vi "GlobalVaribleUnderstanding.vi"() -> ()   [LabVIEW 2019]
uses:
  GlobalVaribleDeclaration.vi
panel:
  out "Your Marks":dbl
  out "Your Full name":string
  out "Are you Marrieed Or not":bool
  out "Age":dbl
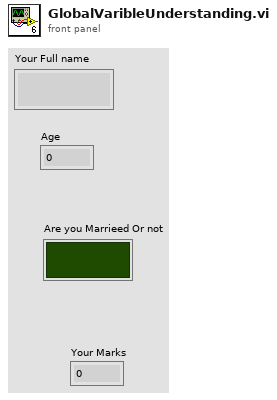
[diagram p1: front panel]
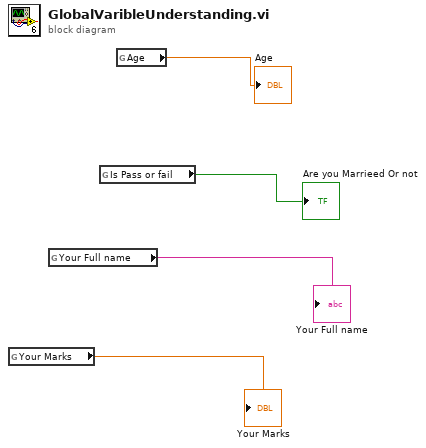
[diagram p0: block diagram]
diagram:
  n1 = global read "GlobalVaribleDeclaration.vi" "Your Marks"() -> (→"Your Marks":dbl)
  n2 = global read "GlobalVaribleDeclaration.vi" "Your Full name"() -> (→"Your Full name":string)
  n3 = global read "GlobalVaribleDeclaration.vi" "Is Pass or fail"() -> (→"Are you Marrieed Or not":bool)
  n4 = global read "GlobalVaribleDeclaration.vi" "Age"() -> (→"Age":dbl)
